vi "Disconnected.vi"(8 "error in (no error)":errorcluster, 11 "TranslationStageUI.lvclass":refnum<class "TranslationStageUI.lvclass">) -> (0 "error out":errorcluster, 3 "TranslationStageUI.lvclass":refnum<class "TranslationStageUI.lvclass">)   [LabVIEW 2023, in "TranslationStage_UI.lvlib" / "TranslationStageUI.lvclass"]
uses:
  TranslationStageUI.lvclass
  TranslationStageUI.lvclass/TranslationStageUI.ctl
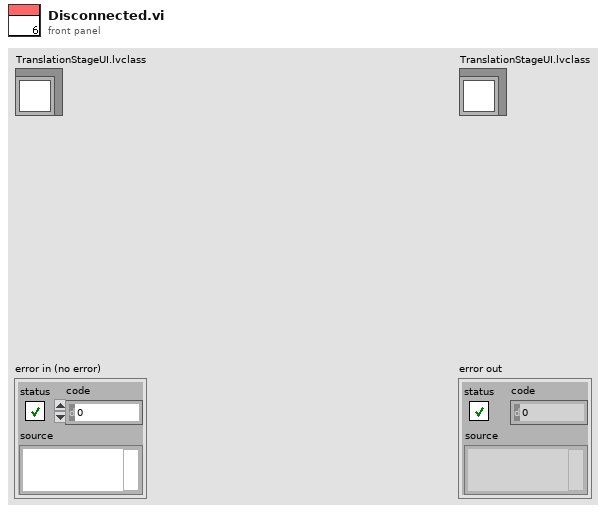
[diagram p1: front panel]
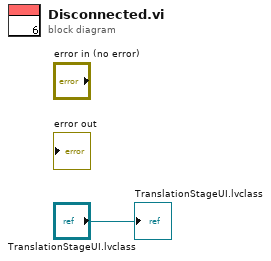
[diagram p0: block diagram]
diagram:
  "TranslationStageUI.lvclass" <- "TranslationStageUI.lvclass"
